vi "Init.vi"(8 "error in":errorcluster, 11 "object in":refnum<class "Continuous Waveform Acq CFG.lvclass">) -> (0 "error out":errorcluster, 3 "object out":refnum<class "Continuous Waveform Acq CFG.lvclass">)   [LabVIEW 2023, in "Continuous Waveform Acq CFG.lvclass"]
uses:
  Continuous Waveform Acq CFG.lvclass
  E:/git/HAL/Scope VISA/Configuration/Scope VISA CFG.lvclass
  HAL/Scope VISA/Configuration/Scope VISA CFG.lvclass/Scope VISA CFG.ctl
  HAL/Scope VISA/Configuration/Scope VISA CFG.lvclass
panel:
  out "Instrument ID":string
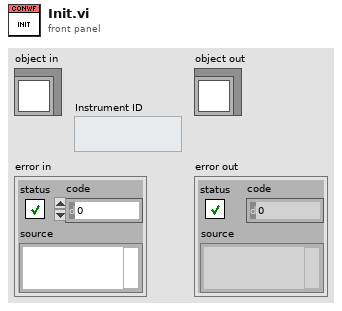
[diagram p1: front panel]
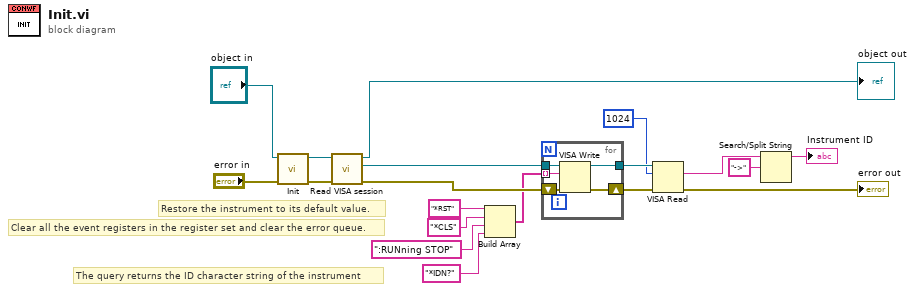
[diagram p0: block diagram]
diagram:
  # "The query returns the ID character string of the instrument"
  # "Clear all the event registers in the register set and clear the error queue."
  # "Restore the instrument to its default value."
  n1 = call-parent "Init.vi"("error in"="error in", "Scope VISA CFG in"="object in") -> ("error out"=w19:errorcluster, "Scope VISA CFG out"=w16:refnum<class "Continuous Waveform Acq CFG.lvclass">)  [unwired: 8 in]
  n2 = call "Read VISA session.vi"("error in (no error)"=w19, "Scope VISA CFG in"=w16) -> ("error out"=w14:errorcluster, "VISA session"=w1:refnum<visa-resource-name>, "Scope VISA CFG out"=→"object out":refnum<class "Continuous Waveform Acq CFG.lvclass">)  [unwired: 7 in]
  n3 = Build Array("*RST", "*CLS" ("write buffer"), ":RUNning STOP" ("element"), "*IDN?") -> (w13:string[])
  n4 = for {
    tunnel: w1 -> [w23]
    tunnel: w13 -> [w22] mode=indexing
    shift-right: [w21] -> w9
    shift-left: w14 -> [w24]
    tunnel: [w20] -> w4
    n5 = VISA Write(VISA resource name=w23, write buffer=w22, error in (no error)=w24) -> (VISA resource name out=w20:refnum<visa-resource-name>, error out=w21:errorcluster)  [unwired: 1 out]
  }
  n6 = VISA Read(VISA resource name=w4, byte count=u32 1024, error in (no error)=w9) -> (read buffer=w7:string, error out=→"error out":errorcluster)  [unwired: 2 out]
  n7 = Search/Split String(string=w7, search string/char (-)="->") -> (substring before match=→"Instrument ID":string)  [unwired: 1 in, 2 out]
